vi "Parametry_AIDI_z_INI_do_tablicy.vi"(7 "Sections in":string[](array[string]), 8 "error in (no error)":errorcluster, 11 "Refnum in":T1) -> (0 "error out":errorcluster, 3 "Refnum out":T1, 4 "Keys out":string[][](array[string]))   [LabVIEW 2014]
doc: "Wczytuje wartoœci kluczy z zadanych sekcji\nw postaci tablicy typu String"
uses:
  <vilib>/Utility/config.llb/Config Data RefNum.ctl
  <vilib>/Utility/config.llb/Read Key (String).vi
  <vilib>/Utility/config.llb/NI_LVConfig.lvlib
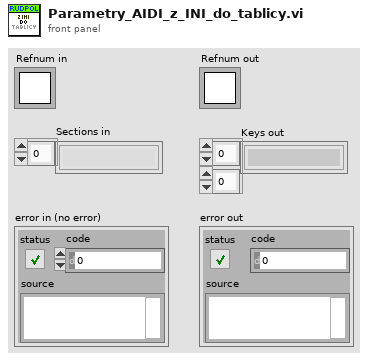
[diagram p1: front panel]
types:
  T1 = typedef "NI_LVConfig.lvlib/Config Data RefNum.ctl" = refnum<k1>
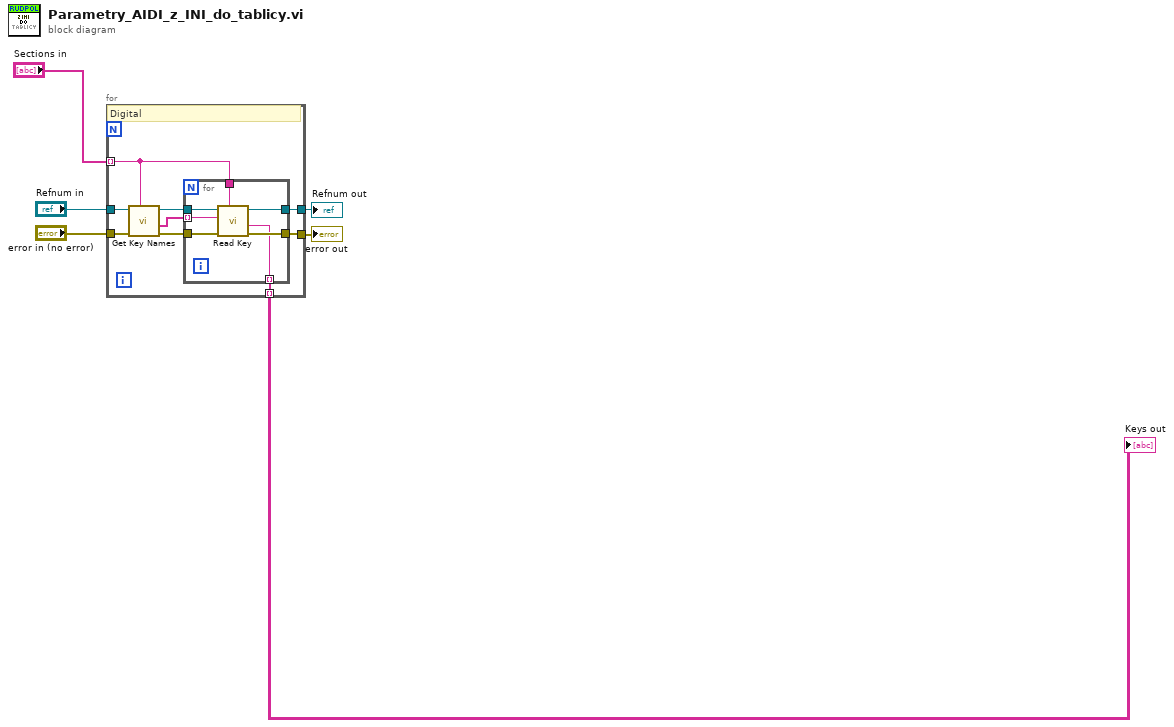
[diagram p0: block diagram]
diagram:
  n1 = for {
    tunnel: "Refnum in" -> [w15]
    tunnel: "error in (no error)" -> [w14]
    tunnel: "Sections in" -> [w10] mode=indexing
    tunnel: [w9] -> w6 mode=indexing
    tunnel: [w8] -> w5
    tunnel: [w7] -> w4
    # "Digital"
    n2 = call <vilib>:"Get Key Names.vi"("section"=w10, "error in (no error)"=w14, "refnum"=w15) -> ("error out"=w12:errorcluster, "key names"=w11:string[], "refnum out"=w13:T1)  [unwired: 5 in, 1 out]
    n3 = for {
      tunnel: w13 -> [w22]
      tunnel: w12 -> [w21]
      tunnel: w11 -> [w20] mode=indexing
      tunnel: w10 -> [w19]
      tunnel: [w18] -> w8
      tunnel: [w17] -> w7
      tunnel: [w16] -> w9 mode=indexing
      n4 = call-poly <vilib>:"Read Key.vi"("section"=w19, "error in (no error)"=w21, "key"=w20, "refnum"=w22) -> ("error out"=w17:errorcluster, "value"=w16:string, "refnum out"=w18:T1)  [unwired: 4 in, 1 out]
    }
  }
  "Keys out" <- w6
  "Refnum out" <- w5
  "error out" <- w4
